vi "Animate To Inactivate.vi"(8 "error in (no error)":errorcluster, 11 "Filled Text Fields Actor in":refnum<class "Filled Text Fields Actor.lvclass">) -> (0 "error out":errorcluster, 3 "Filled Text Fields Actor out":refnum<class "Filled Text Fields Actor.lvclass">)   [LabVIEW 2017, in "Filled Text Fields Actor.lvlib" / "Filled Text Fields Actor.lvclass"]
uses:
  Filled Text Fields Actor.lvclass
  Filled Text Fields Actor.lvclass/Filled Text Fields Actor.ctl
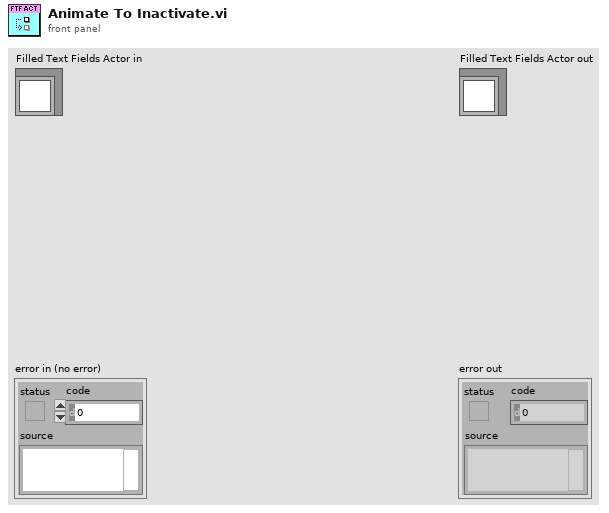
[diagram p1: front panel]
types:
  T1 = typedef "LVPositionTypeDef.ctl" = cluster{"Left":i32, "Top":i32}
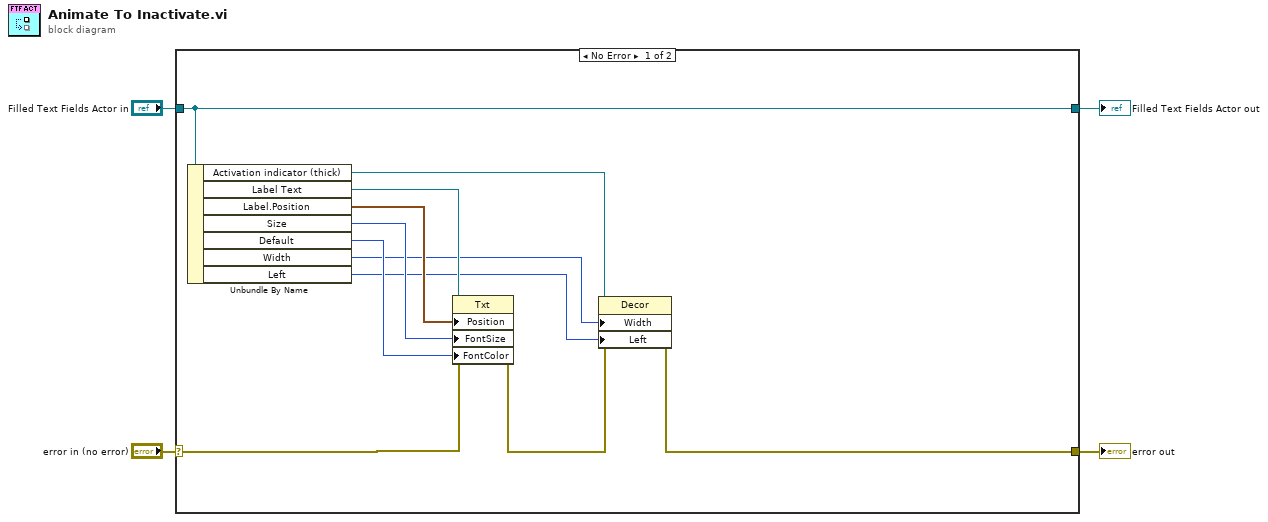
[diagram p0: block diagram]
diagram:
  n1 = case shown="No Error" "error in (no error)" {
    selector: "error in (no error)" -> [w13 w17]
    tunnel: [w7 w17] -> w3
    tunnel: [w15 w16] -> w1
    tunnel: "Filled Text Fields Actor in" -> [w15 w16]
    frame No Error {
      n2 = Unbundle By Name(w15) -> ("Activation indicator (thick)"=w9:refnum<vi>, "Label Text"=w14:refnum<vi>, "Label.Position"=w12:T1, "Size"=w11:u32, "Default"=w10:u32, "Width"=w6:u32, "Left"=w5:i32)
      n3 = property class="Txt"(reference=w14, error in=w13, "Position"=w12, "FontSize"=w11, "FontColor"=w10) -> (error out=w8:errorcluster)  [unwired: 1 out]
      n4 = property class="Decor"(reference=w9, error in=w8, "Width"=w6, "Left"=w5) -> (error out=w7:errorcluster)  [unwired: 1 out]
    }
    frame Error {
    }
  }
  "error out" <- w3
  "Filled Text Fields Actor out" <- w1
